vi "ParGetStat.vi"(0 "ref in":u64, 11 "error in (no error)":errorcluster) -> (2 "Bytes Recv":i32, 3 "Bytes Sent":i32, 4 "ref out":u64, 13 "Send Errors":i32, 14 "Recv Errors":i32, 15 "error out":errorcluster)   [LabVIEW 2018, in "Snap7.lvlib"]
uses:
  Snap7.lvlib
  windows/lv_snap7.dll
panel:
  in  "var RecvErrors":i32
  in  "var SendErrors":i32
  in  "var bytesrecv":i32
  in  "var bytessent":i32
  out "Result":i32
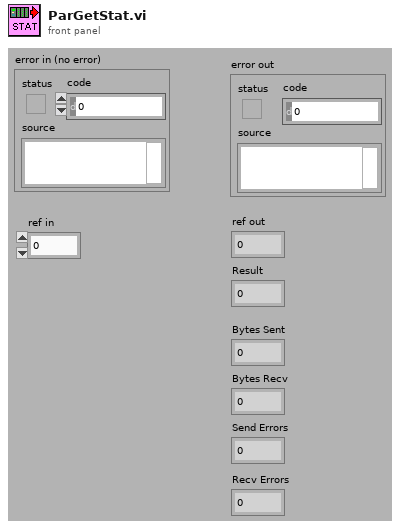
[diagram p1: front panel]
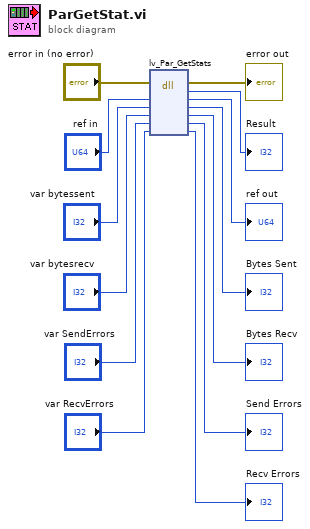
[diagram p0: block diagram]
diagram:
  n1 = dll-call lib="PTH2iabs D项目Feng恒隆项目Labview性能试验台SourcesSnap7libwindowslv_snap7.dll" fn="lv_Par_GetStats"(error in="error in (no error)", "Partner"="ref in", "BytesSent"="var bytessent", "BytesRecv"="var bytesrecv", "SendErrors"="var SendErrors", "RecvErrors"="var RecvErrors") -> (error out=→"error out":errorcluster, "return type"=→"Result":i32, "Partner"=→"ref out":u64, "BytesSent"=→"Bytes Sent":i32, "BytesRecv"=→"Bytes Recv":i32, "SendErrors"=→"Send Errors":i32, "RecvErrors"=→"Recv Errors":i32)  [unwired: 2 in, 1 out]
